vi "wait until btn released.vi"(10 "index":i32, 11 "JoystickDevRef":T1) -> (3 "JoystickDevRef 2":T1)   [LabVIEW 2019]
uses:
  <vilib>/Rock Robotics/WPI/Joystick/WPI_JoystickDevRef.ctl
  <vilib>/Rock Robotics/WPI/Joystick/WPI_JoystickDeviceEnum.ctl
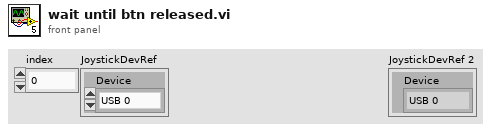
[diagram p1: front panel]
types:
  T1 = typedef "WPI_JoystickDevRef.ctl" = cluster{"Device":T2}
  T2 = typedef "WPI_JoystickDeviceEnum.ctl" = enum16{"USB 0", "USB 1", "USB 2", "USB 3", "USB 4", "USB 5"}
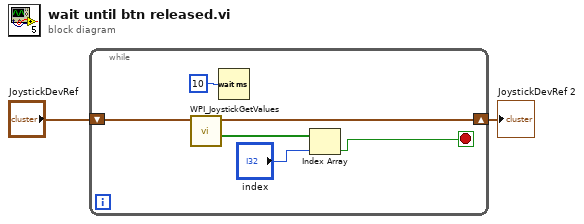
[diagram p0: block diagram]
diagram:
  n1 = while {
    shift-right: [w7] -> w1
    shift-left: "JoystickDevRef" -> [w8]
    stop <- w4 stop-if-true
    n2 = call <vilib>:"WPI_JoystickGetValues.vi"("JoystickDevRef"=w8) -> ("Buttons"=w5:bool[], "JoystickDevRef"=w7:T1)  [unwired: 6 in, 3 out]
    n3 = Wait (ms)(milliseconds to wait=u32 10) -> ()  [unwired: 1 out]
    n4 = Index Array(array=w5, index="index") -> (element=w4:bool)
  }
  "JoystickDevRef 2" <- w1
